vi "Tmp_M Main.vi"(9 "timeout ms":i32=1000, 10 "Queue to master":T2, 11 "Module queue":T2) -> (0 "Error Out":errorcluster, 3 "Temperatures":T1[](array[typedef]) {"Time stamp" format="%<%H:%M:%S%2u\n%Y/%m/%d>T"})   [LabVIEW 2021, in "Magnet module.lvlib"]
doc: "Magnet module controls: power supply unit (PSU/SMS) and temperature monitor (TM/LSC218).\nPSU controls mainly: switch heater and ramping of current which runs throught coil.\nTM controls temperature of switch, coil and cryostat.\nMessage for magnet is a cluster that contains: {(enum) Command , (variant) Data}\nFor simplifieing of documentation, the Command is noted as a name of instruction, and Data is represented by a requered datatype (mostly cluster) name.\nCommands:\nInitialize(Magnet Config Constants) - Sugesstion: Load configuration constants from configuration file.\nSet field (Set field{B, R, cr}) - B-field[T], R-ramp[A/s], cr - custom ramp[bool].\nSwitch mode(mode) - to persistant, or to ramping.\nBlackout() - undone functionality of emergency deenergizing.\nUpdate() - Important! This triggers update of data from instruments. Shoud occure in regular intervals as priority message.\nResponses:\nMagnet initialized ();\nTM revision(temperature monitor revision);\nMagnet init error(error);\nSetting field(Set Field{B, R, cr});\nWarning(string);\nSwitching to(mode);\nUpdate error(error);\nTM update(TM sensors);\nPSU update(PSU data);\nMagnet status();"
uses:
  Magnet module.lvlib
  Messenger service/Data types/Mailbox address.ctl
  ctl/Cryostat temperature sensors.ctl
  Messenger service/Data types/Module name.ctl
  Messenger service/MessengerLib.lvlib
panel:
  out "Connected":bool
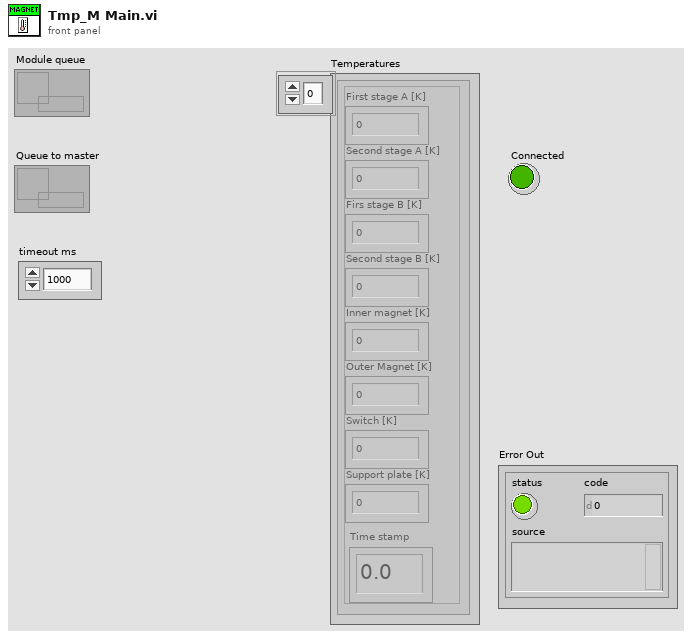
[diagram p1: front panel]
types:
  T1 = typedef "Magnet module.lvlib/Cryostat temperature sensors.ctl" = cluster{"First stage A [K]":dbl, "Second stage A [K]":dbl, "Firs stage B [K]":dbl, "Second stage B [K]":dbl, "Inner magnet [K]":dbl, "Outer Magnet [K]":dbl, "Switch [K]":dbl, "Support plate [K]":dbl, "Time stamp":dbl}
  T2 = typedef "MessengerLib.lvlib/Mailbox address.ctl" = refnum<queue>
  T3 = typedef "Module name.ctl" = enum16{"Emty", "Magnet", "VTI", "Excitation", "Servo", "Acquisition", "Rotator", "Digitizer", "SMU2450", "Carousel", "Multimeter", "Tmp monitor", "Power monitor"}
  T4 = typedef "Magnet module.lvlib/Tmp_M commands.ctl" = enum16{"Ignore", "Connect", "Set timeout", "Update", "Disconnect"}
  T5 = typedef "Magnet module.lvlib/TM Revision.ctl" = cluster{"Instr Serial Number":string, "Instr Driver Revision":string, "Instr Firmware Revision":string, "Instr Model Number":string}
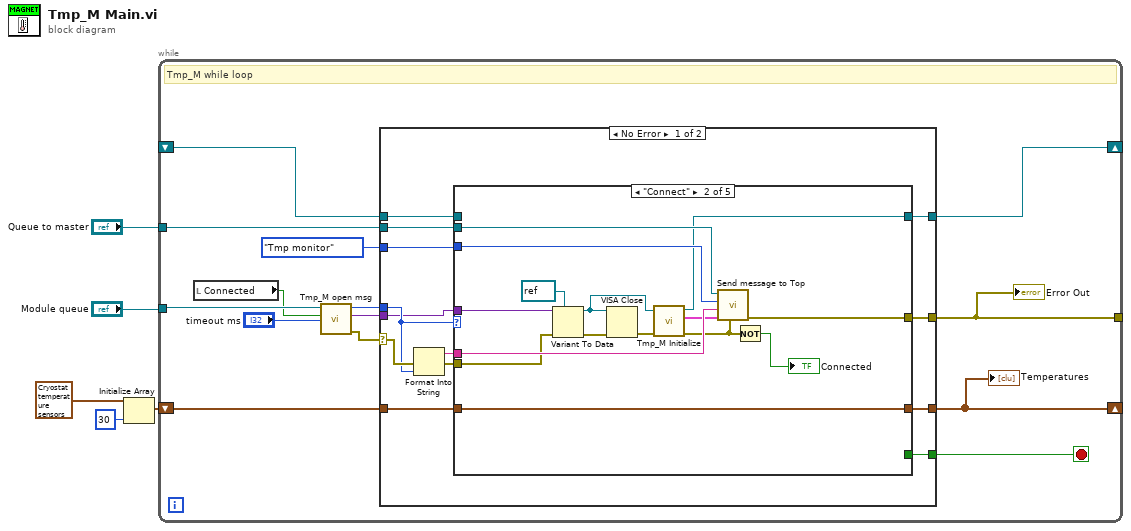
[diagram p0: block diagram]
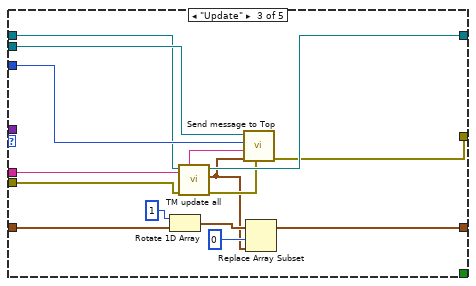
[diagram p3: hidden frame]
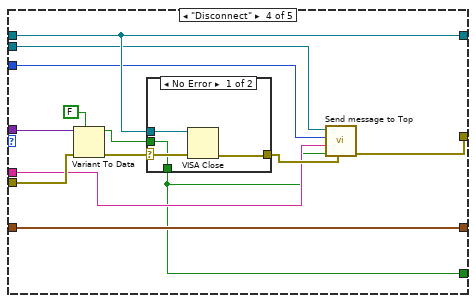
[diagram p4: hidden frame]
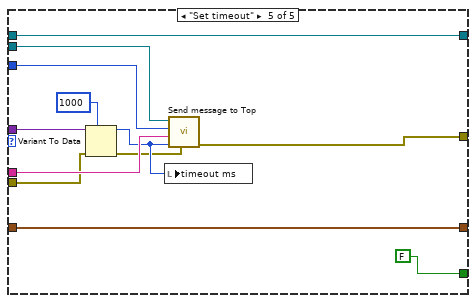
[diagram p6: hidden frame]
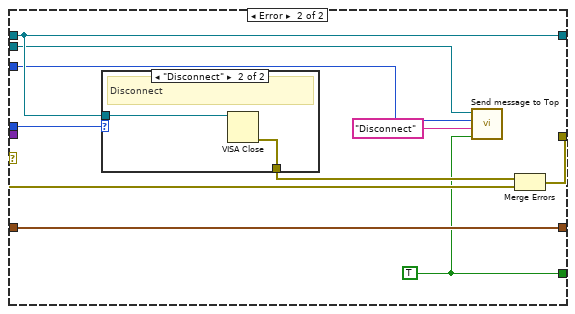
[diagram p7: hidden frame]
diagram:
  n1 = Initialize Array(T1 {"First stage A [K]"=0.0, "Second stage A [K]"=0.0, "Firs stage B [K]"=0.0, "Second stage B [K]"=0.0, "Inner magnet [K]"=0.0, "Outer Magnet [K]"=0.0, "Switch [K]"=0.0, "Support plate [K]"=0.0, "Time stamp"=0.0} ("LSC218 sensors"), 30 ("dimension size")) -> (w3:T1[])
  n2 = while {
    tunnel: "Module queue" -> [w14]
    tunnel: "Queue to master" -> [w19]
    shift-right: [w17] -> _
    shift-left: w3 -> [w18]
    shift-right: [w16] -> _
    shift-left: _ -> [w15]
    tunnel: [w6] -> _
    stop <- w10 stop-if-true
    # "Tmp_M while loop"
    n3 = local read "Connected"() -> (w7:bool)
    n4 = call "Tmp_M open msg.vi"("timeout ms (1000)"="timeout ms", "Connected"=w7, "Queue in"=w14) -> ("error out"=w12:errorcluster, "Data"=w11:variant, "Command"=w13:T4)  [unwired: 4 in, 2 out]
    n5 = case shown="No Error" w12 {
      selector: w12 -> [w25 w99]
      tunnel: w19 -> [w32 w97]
      tunnel: w13 -> [w24 w103]
      tunnel: w18 -> [w31 w104]
      tunnel: [w30 w104] -> w17
      tunnel: [w21 w95] -> w10
      tunnel: [w28 w102] -> w16
      tunnel: w15 -> [w27 w102]
      tunnel: w11 -> [w23 _]
      tunnel: [w22 w101] -> w6
      tunnel: Module_name."Tmp monitor" ("Module") -> [w20 w98]
      frame No Error {
        n6 = Format Into String(error in=w25, w24) -> (resulting string=w29:string, error out=w26:errorcluster)  [unwired: 2 in]
        n7 = case shown="\"Connect\"" w24 {
          tunnel: w32 -> [_ w50 w60 w69 w93]
          tunnel: w31 -> [w35 w49 w64 w77 w94]
          tunnel: [w35 w49 w63 w77 w94] -> w30
          tunnel: w20 -> [_ w46 w61 w68 w90]
          tunnel: w29 -> [_ w47 w62 w67 w91]
          tunnel: [_ _ _ w65 FALSE] -> w21
          tunnel: [w34 w43 w58 w76 w89] -> w28
          tunnel: w27 -> [w34 _ w59 w76 w89]
          tunnel: w26 -> [w33 w39 w51 w73 w86]
          tunnel: w23 -> [_ w38 _ w74 w87]
          tunnel: [w33 w37 w57 w70 w83] -> w22
          frame "Ignore", Default {
          }
          frame "Connect" {
            n8 = Variant To Data(error in=w39, type=refnum<visa-resource-name> refnum ("LSC218"), Variant=w38) -> (data=w42:refnum<visa-resource-name>, error out=w48:errorcluster)
            n9 = VISA Close(VISA resource name=w42, error in (no error)=w48) -> (error out=w45:errorcluster)
            n10 = call "Tmp_M Initialize.vi"("error in (no error)"=w45, "VISA Refnum in"=w42) -> ("error out"=w40:errorcluster, "TM Revision"=w44:T5, "VISA Refnum out"=w43:refnum<visa-resource-name>)  [unwired: 7 in]
            n11 = call "Send message to Top.vi"("Error in (no error)"=w40, "Data"=w44, "Response"=w47, "Module"=w46, "Mailbox address in"=w50) -> ("Error out"=w37:errorcluster)  [unwired: 5 in, 1 out]
            n12 = Not(x=w40) -> (.not. x?=→"Connected":bool)
          }
          frame "Update" {
            n13 = Rotate 1D Array(1:w64, 2:1 ("n")) -> (0:w55:T1[])
            n14 = call "TM update all.vi"("error in (no error)"=w51, "VISA Refnum in"=w59) -> ("error out"=w53:errorcluster, "LSC218 sensors"=w52:T1, "VISA Refnum out"=w58:refnum<visa-resource-name>)  [unwired: 7 in]
            n15 = call "Send message to Top.vi"("Error in (no error)"=w53, "Data"=w52, "Response"=w62, "Module"=w61, "Mailbox address in"=w60) -> ("Error out"=w57:errorcluster)  [unwired: 5 in, 1 out]
            n16 = Replace Array Subset(array=w55, new element=w52, index=0) -> (w63:T1[])
          }
          frame "Disconnect" {
            n17 = Variant To Data(error in=w73, type=FALSE, Variant=w74) -> (data=w66:bool, error out=w72:errorcluster)
            n18 = case shown="No Error" w72 {
              selector: w72 -> [w80 w82]
              tunnel: w76 -> [w81 _]
              tunnel: [w79 w82] -> w71
              tunnel: w66 -> [w78 _]
              tunnel: [w78 _] -> w65
              frame No Error {
                n19 = VISA Close(VISA resource name=w81, error in (no error)=w80) -> (error out=w79:errorcluster)
              }
              frame Error {
              }
            }
            n20 = call "Send message to Top.vi"("Error in (no error)"=w71, "Data"=w65, "Response"=w67, "Module"=w68, "Mailbox address in"=w69) -> ("Error out"=w70:errorcluster)  [unwired: 5 in, 1 out]
          }
          frame "Set timeout" {
            n21 = Variant To Data(error in=w86, type=1000 ("timeout ms"), Variant=w87) -> (data=w85:i32, error out=w84:errorcluster)
            n22 = local write "timeout ms"(w85) -> ()
            n23 = call "Send message to Top.vi"("Error in (no error)"=w84, "Data"=w85, "Response"=w91, "Module"=w90, "Mailbox address in"=w93) -> ("Error out"=w83:errorcluster)  [unwired: 5 in, 1 out]
          }
        }
      }
      frame Error {
        w95 = TRUE
        n24 = case shown="\"Disconnect\"" w103 {
          tunnel: w102 -> [_ w106]
          tunnel: [_ w105] -> w100
          frame "Ignore", Default {
            # "Nohing"
          }
          frame "Disconnect" {
            # "Disconnect"
            n25 = VISA Close(VISA resource name=w106) -> (error out=w105:errorcluster)  [unwired: 1 in]
          }
        }
        n26 = call "Send message to Top.vi"("Data"=w95, "Response"="Disconnect", "Module"=w98, "Mailbox address in"=w97) -> ()  [unwired: 6 in, 2 out]
        n27 = Merge Errors(w100, w99) -> (w101:errorcluster)
      }
    }
    "Temperatures" <- w17
    "Error Out" <- w6
  }
